vi "datahandle.vi"(0 "object in":refnum<class "tcp_work.lvclass">, 1 "字符串":string, 5 "error in (no error)":errorcluster) -> (14 "object out":refnum<class "tcp_work.lvclass">, 15 "命令编码CN":string, 16 "时间QN":string, 17 "数据":string, 18 "布尔":bool, 19 "error out":errorcluster)   [LabVIEW 2016, in "tcp_work.lvclass"]
uses:
  tcp_work.lvclass
panel:
  out "拆分包及应答Flag":string
  out "设备编码MN":string
  out "密码PW":string
  out "系统编码ST":string
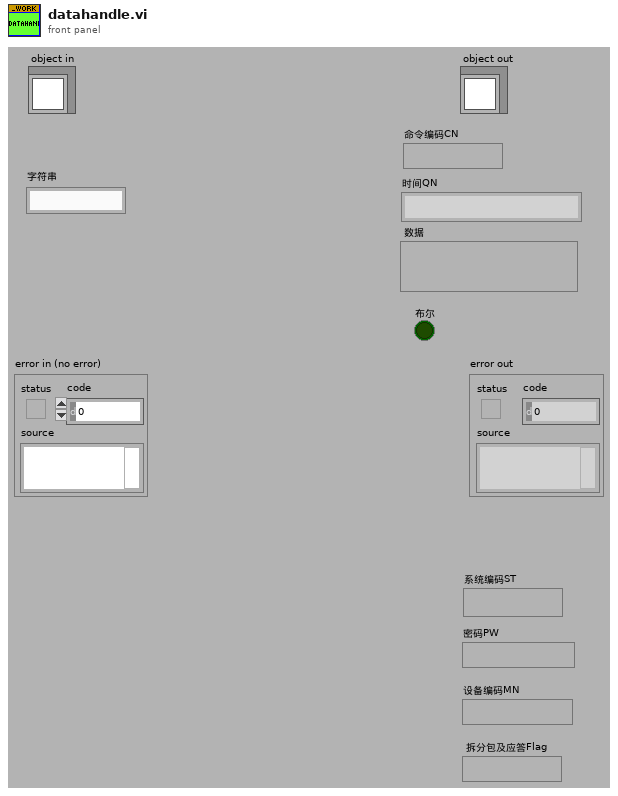
[diagram p1: front panel]
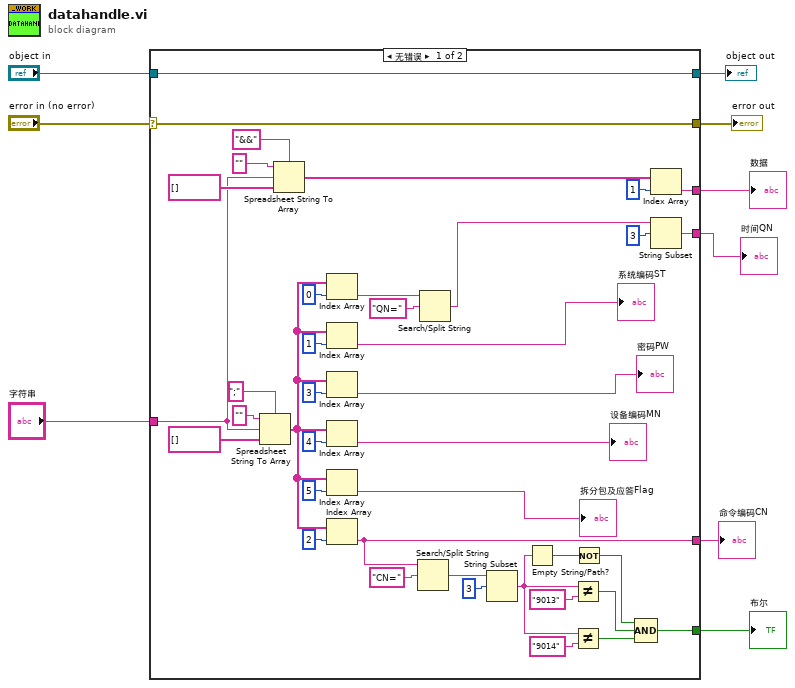
[diagram p0: block diagram]
diagram:
  n1 = case shown="无错误" "error in (no error)" {
    selector: "error in (no error)" -> [w49 w51]
    tunnel: [w49 w51] -> w8
    tunnel: [w48 w50] -> w6
    tunnel: "object in" -> [w48 w50]
    tunnel: "字符串" -> [w28 _]
    tunnel: [w17 _] -> w4
    tunnel: [w16 _] -> w3
    tunnel: [w15 _] -> w2
    tunnel: [w10 _] -> w1
    frame No Error {
      n2 = Spreadsheet String To Array(delimiter (Tab)=";" ("分隔符(Tab)"), format string="" ("格式字符串"), spreadsheet string=w28, array type (2D Dbl)=string[] [] ("数组")) -> (array=w32:string[])
      n3 = Spreadsheet String To Array(delimiter (Tab)="&&" ("分隔符(Tab)"), format string="" ("格式字符串"), spreadsheet string=w28, array type (2D Dbl)=string[] [] ("数组")) -> (array=w46:string[])
      n4 = Index Array(array=w32, index=0 ("索引")) -> (element=w11:string)
      n5 = Index Array(array=w32, index=1 ("索引")) -> (element=→"系统编码ST":string)
      n6 = Index Array(array=w32, index=3 ("索引")) -> (element=→"密码PW":string)
      n7 = Index Array(array=w32, index=4 ("索引")) -> (element=→"设备编码MN":string)
      n8 = Index Array(array=w32, index=5 ("索引")) -> (element=→"拆分包及应答Flag":string)
      n9 = Index Array(array=w32, index=2 ("索引")) -> (element=w15:string)
      n10 = Search/Split String(string=w15, search string/char (-)="CN=" ("搜索字符串/字符(-)")) -> (match + rest of string=w25:string)  [unwired: 1 in, 2 out]
      n11 = Search/Split String(string=w11, search string/char (-)="QN=" ("搜索字符串/字符(-)")) -> (match + rest of string=w12:string)  [unwired: 1 in, 2 out]
      n12 = String Subset(string=w25, offset (0)=3 ("偏移量(0)")) -> (substring=w23:string)  [unwired: 1 in]
      n13 = Empty String/Path?(string/path=w23) -> (empty?=w24:bool)
      n14 = Not Equal?(x=w23, y="9013") -> (x != y?=w20:bool)
      n15 = Not Equal?(x=w23, y="9014") -> (x != y?=w19:bool)
      n16 = Not(x=w24) -> (.not. x?=w18:bool)
      n17 = Compound Arithmetic op=AND ("复合运算")(w18, w20, w19) -> (w17:bool)
      n18 = Index Array(array=w46, index=1 ("索引")) -> (element=w16:string)
      n19 = String Subset(string=w12, offset (0)=3 ("偏移量(0)")) -> (substring=w10:string)  [unwired: 1 in]
    }
    frame Error {
    }
  }
  "error out" <- w8
  "object out" <- w6
  "布尔" <- w4
  "数据" <- w3
  "时间QN" <- w1
  "命令编码CN" <- w2
